vi "generate_DAC_voltages_galvo.vi"(8 "derived values":T1, 10 "counter cluster in":T2, 11 "resonant trigger":bool) -> (0 "acquire?":bool, 1 "fly-back acquisition phase?":bool, 2 "counter cluster out":T2)   [LabVIEW 2010]
uses:
  type definitions/counter_cluster.ctl
  type definitions/derived_values_cluster.ctl
panel:
  in  "x offset fly-forward (iterations)":u16
  out "x .or. y?":bool
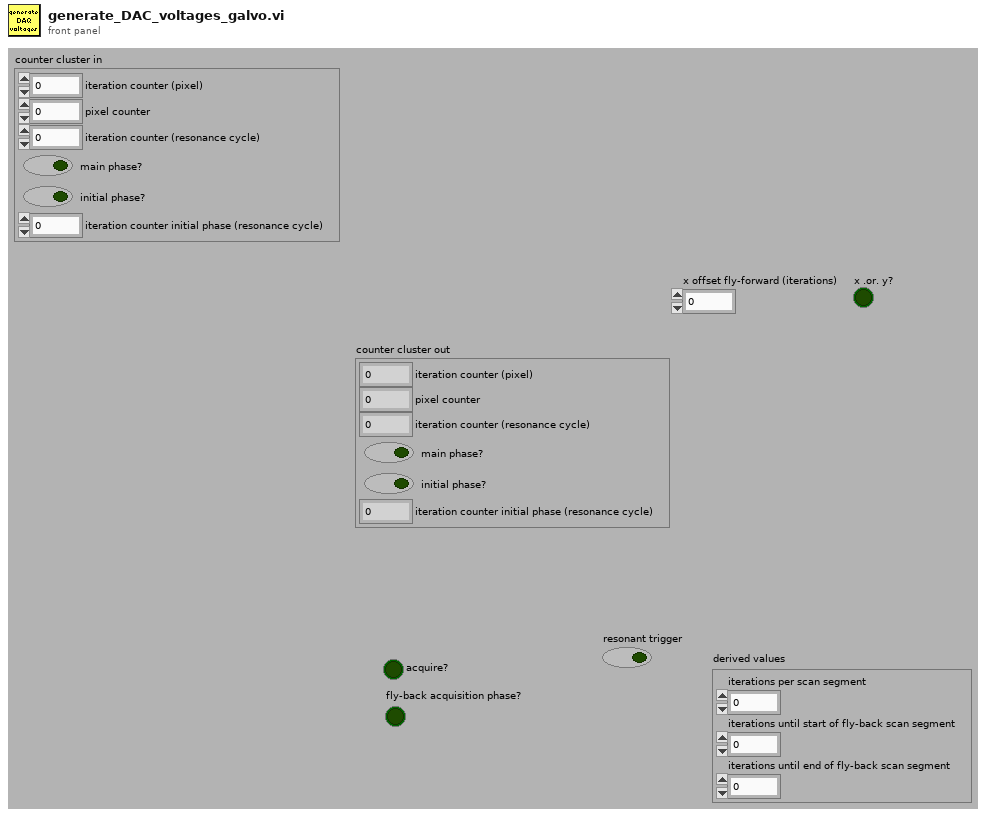
[diagram p1: front panel]
types:
  T1 = typedef "derived_values_cluster.ctl" = cluster{"iterations per scan segment":u16, "iterations until start of fly-back scan segment":u16, "iterations until end of fly-back scan segment":u16}
  T2 = typedef "counter_cluster.ctl" = cluster{"iteration counter (pixel)":u16, "pixel counter":u16, "iteration counter (resonance cycle)":u16, "main phase?":bool, "initial phase?":bool, "iteration counter initial phase (resonance cycle)":u16}
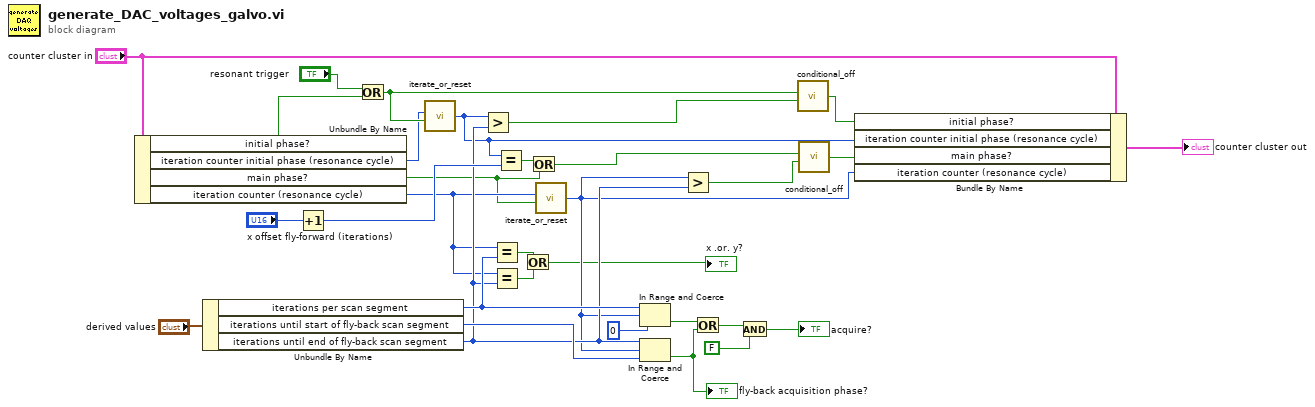
[diagram p0: block diagram]
diagram:
  n1 = Unbundle By Name("counter cluster in") -> ("initial phase?"=w26:bool, "iteration counter initial phase (resonance cycle)"=w7:u16, "main phase?"=w6:bool, "iteration counter (resonance cycle)"=w12:u16)
  n2 = Unbundle By Name("derived values") -> ("iterations per scan segment"=w24:u16, "iterations until start of fly-back scan segment"=w27:u16, "iterations until end of fly-back scan segment"=w16:u16)
  n3 = Increment(x="x offset fly-forward (iterations)") -> (x+1=w18:u16)
  n4 = Or(x="resonant trigger", y=w26) -> (x .or. y?=w21:bool)
  n5 = call "iterate_or_reset.vi"("iterate?"=w21, "number in"=w7) -> ("number out"=w5:u16)  [unwired: 4 in]
  n6 = Greater?(x=w5, y=w16) -> (0:w17:bool)
  n7 = Equal?(x=w12, y=w24) -> (x = y?=w14:bool)
  n8 = Equal?(x=w12, y=w16) -> (x = y?=w15:bool)
  n9 = Equal?(x=w5, y=w18) -> (x = y?=w22:bool)
  n10 = Or(x=w14, y=w15) -> (x .or. y?=→"x .or. y?":bool)
  n11 = Or(x=w22, y=w6) -> (x .or. y?=w4:bool)
  n12 = call "iterate_or_reset.vi"("iterate?"=w6, "number in"=w12) -> ("number out"=w13:u16)  [unwired: 4 in]
  n13 = In Range and Coerce(upper limit=w24, x=w13, lower limit=u16 0) -> (In Range?=w30:bool)  [unwired: 1 out]
  n14 = In Range and Coerce(upper limit=w16, x=w13, lower limit=w27) -> (In Range?=w9:bool)  [unwired: 1 out]
  "fly-back acquisition phase?" <- w9
  n15 = Greater?(x=w13, y=w16) -> (0:w3:bool)
  n16 = Or(x=w30, y=w9) -> (x .or. y?=w29:bool)
  n17 = And(x=w29, y=FALSE) -> (x .and. y?=→"acquire?":bool)
  n18 = call "conditional_off.vi"("switch off?"=w17, "boolean in"=w21) -> ("boolean out"=w20:bool)  [unwired: 4 in]
  n19 = call "conditional_off.vi"("switch off?"=w3, "boolean in"=w4) -> ("boolean out"=w19:bool)  [unwired: 4 in]
  n20 = Bundle By Name(cluster="counter cluster in", "initial phase?"=w20, "iteration counter initial phase (resonance cycle)"=w5, "main phase?"=w19, "iteration counter (resonance cycle)"=w13) -> (→"counter cluster out":T2)
